vi "Launch Helper Loop.vi"(8 "error in (no error)":errorcluster, 9 "Message Data":variant, 10 "Message":string, 11 "Helper Loop In":refnum<class "Helper Loop.lvclass">) -> (0 "error out":errorcluster, 3 "Helper Loop Out":refnum<class "Helper Loop.lvclass">)   [LabVIEW 2020, in "Helper Loop.lvclass"]
doc: "Launches an asynchronous helper loop. Multiple helper loops may be launched using multiple calls to this VI. The Message and Message Data provided to this VI will be available in the Helper Action.vi once running."
uses:
  Helper Loop.lvclass
  Process/Process.lvclass
  <vilib>/ErrorRing/Error Ring.xnode
  <vilib>/Utility/error.llb/Error Cluster From Error Code.vi
  Process/Public/Lifecycle/API Mode.ctl
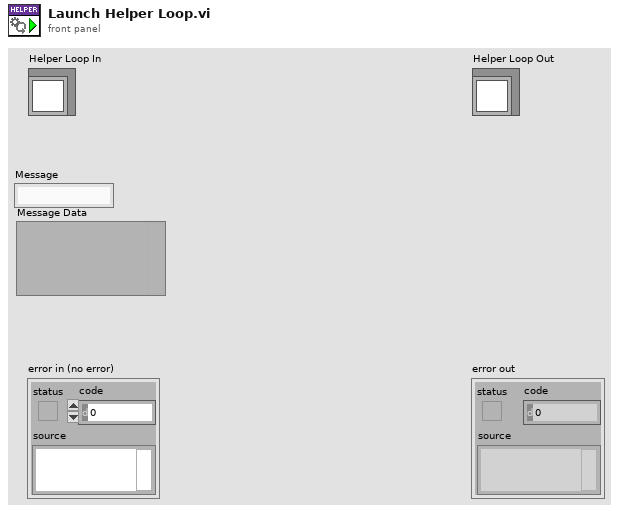
[diagram p1: front panel]
types:
  T1 = typedef "Process.lvclass/API Mode.ctl" = enum16{"Send Message", "Handle Message"}
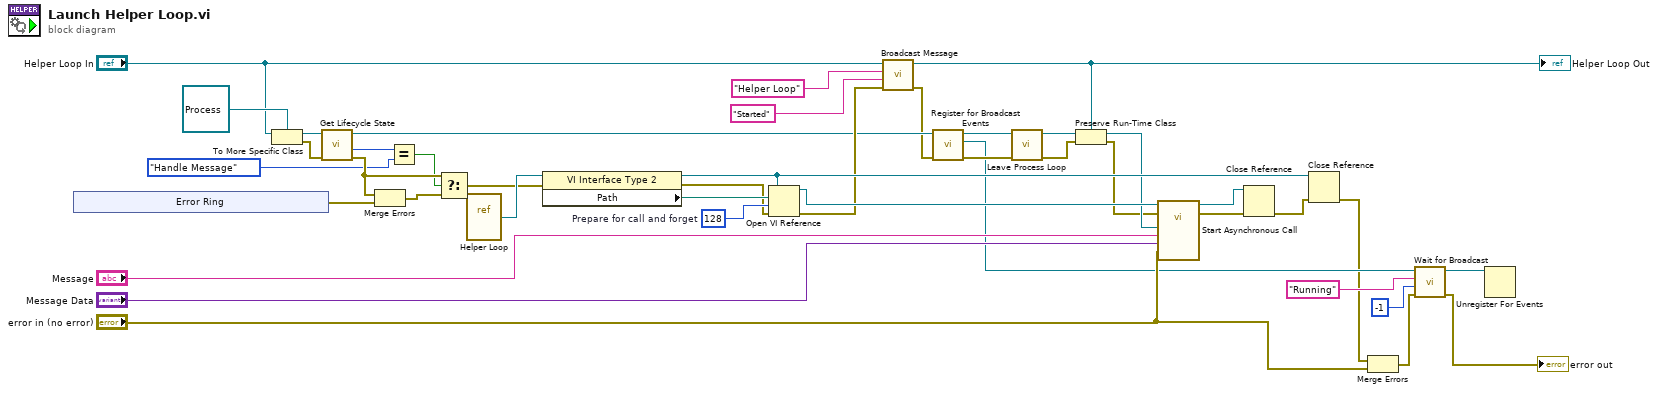
[diagram p0: block diagram]
diagram:
  w37 = 128  # Prepare for call and forget
  n1 = xnode "Error Ring"() -> ("error out"=w22:errorcluster)
  n2 = To More Specific Class(target class=refnum<class "Process.lvclass"> refnum ("Process Out"), reference="Helper Loop In") -> (specific class reference=w31:refnum<class "Process.lvclass">, error out=w26:errorcluster)  [unwired: 1 in]
  n3 = call "Get Lifecycle State.vi"("error in (no error)"=w26, "Process In"=w31) -> ("error out"=w25:errorcluster, "API Mode"=w24:T1, "Process Out"=w27:refnum<class "Process.lvclass">)  [unwired: 6 in, 1 out]
  n4 = Merge Errors(w25, w22) -> (w23:errorcluster)
  n5 = Equal?(x=w24, y=API_Mode."Handle Message") -> (x = y?=w2:bool)
  n6 = Select(t=w25, s=w2, f=w23) -> (s? t:f=w20:errorcluster)
  n7 = vi-ref "Helper Loop.vi"() -> (w38:refnum<vi>)
  n8 = property class="VI Interface Type 2"(reference=w38, error in=w20) -> (reference out=w32:refnum<vi>, error out=w34:errorcluster, "Path"=w35:path)
  n9 = Open VI Reference(type specifier VI Refnum (for type only)=w32, vi path=w35, options=w37, error in (no error)=w34) -> (vi reference=w36:refnum<vi>, error out=w28:errorcluster)  [unwired: 2 in]
  n10 = call-dynamic "Broadcast Message.vi"("error in (no error)"=w28, "Message Data"="Started", "Message"="Helper Loop", "Helper Loop in"="Helper Loop In") -> ("error out"=w15:errorcluster, "Helper Loop out"=w16:refnum<class "Helper Loop.lvclass">)  [unwired: 6 in]
  "Helper Loop Out" <- w16
  n11 = call "Register for Broadcast Events.vi"("error in (no error)"=w15, "Process In"=w27) -> ("error out"=w18:errorcluster, "Event Registration Refnum Out"=w12:refnum<event-registration>, "Process Out"=w4:refnum<class "Process.lvclass">)  [unwired: 7 in]
  n12 = call "Leave Process Loop.vi"("error in (no error)"=w18, "Process In"=w4) -> ("error out"=w5:errorcluster, "Process Out"=w3:refnum<class "Process.lvclass">)  [unwired: 8 in]
  n13 = Preserve Run-Time Class(object in=w3, error in=w5, 2:w16) -> (object out=w30:refnum<class "Helper Loop.lvclass">, error out=w19:errorcluster)
  n14 = call-by-ref "Start Asynchronous Call"(reference=w36, error in=w19, 8:"error in (no error)"="error in (no error)", "Message Data"="Message Data", "Message"="Message", "Helper Loop In"=w30) -> (reference out=w40:refnum<vi>, error out=w39:errorcluster)  [unwired: 6 in, 2 out]
  n15 = Close Reference(reference=w40, error in (no error)=w39) -> (error out=w33:errorcluster)
  n16 = Close Reference(reference=w32, error in (no error)=w33) -> (error out=w8:errorcluster)
  n17 = Merge Errors(w8, "error in (no error)") -> (w7:errorcluster)
  n18 = call "Wait for Broadcast.vi"("error in (no error)"=w7, "Timeout [ms]"=-1 ("Loop Period [ms]"), "Broadcast Message"="Running", "Event Registration Refnum in"=w12) -> ("error out"=→"error out":errorcluster, "Event Registration Refnum out"=w11:refnum<event-registration>)  [unwired: 5 in, 1 out]
  n19 = Unregister For Events(event registration refnum=w11) -> ()  [unwired: 1 in, 1 out]
